vi "OutputSwerveDrive.vi"() -> ()   [LabVIEW 2020]
doc: "This VI runs feedback and feedforward controllers, manages safety interlocks, and sends commands to the swerve drive motors. This VI also controls the commanded drive shifter (low gear or high gear) state."
uses:
  <vilib>/Rock Robotics/WPI/DriverStation/WPI_DriverStationRobotMode2.ctl
  <vilib>/Rock Robotics/WPI/Solenoid/WPI_SolenoidValue.ctl
  <vilib>/Rock Robotics/WPI/ThirdParty/Phoenix-LabVIEW/Motor Controller/Controls/CTRE_Phoenix_MotorControl_ControlMode.ctl
  <vilib>/Rock Robotics/WPI/ThirdParty/Phoenix-LabVIEW/Motor Controller/Controls/CTRE_Phoenix_MotorControl_NeutralMode.ctl
  9914bed3-0d1c-4b06-b050-22aab9a27a8c.vi
  21d1f6ed-8aa7-4c08-a7f4-4e12b9ae70b2.vi
  bd7bff45-d105-4c72-b52f-b7d898b15bf8.vi
  96bdb372-2377-4471-891f-ae36cd8cf6e7.vi
  4a6563c0-2600-4cc4-b814-5bfdd37bee33.vi
  59edaa1e-6d55-4e0d-9ccd-6771bdd34e38.vi
  9422521f-1ab3-4d1d-a0e1-edf0c1a6602b.vi
  164a13db-b17b-4981-8c2b-304dea5fbafc.vi
  bf4fe2dc-b12c-4808-b801-08a1d6a94233.vi
  dd2354c2-df0e-4340-ba82-09bb2e9cf5c3.vi
  13dda775-fe22-4909-989b-e16af49b0f34.vi
  2fe6b0e9-d121-4a66-8d55-455f8b7e1020.vi
  e77e916c-e179-4e89-92bf-a3cab155e43b.vi
  sensordata.vi
  robotoutputs.vi
  GlobalDriverStationData.vi
  GlobalAutonomous.vi
  GlobalDrivebase.vi
  GRNF_CTREMotor.vi
  <vilib>/Rock Robotics/WPI/ThirdParty/Phoenix-LabVIEW/Motor Controller/Get/CTRE_Phoenix_MotorController_GetSelectedSensorData.vi
  TAI_Solenoid.vi
  GRNF_GenericSolenoid.vi
  <vilib>/Rock Robotics/WPI/Solenoid/WPI_SolenoidSetEnum.vi
  TAI_Motor.vi
panel:
  in  "Slew Rate When Slow (/s)":dbl=1.0
  in  "Slew Rate When Fast (/s)":dbl=0.8
  in  "Force to Low Gear":bool
  in  "Force To High Gear":bool
  in  "Drive Command Override [0,1]":dbl min=0.0 max=1.0 step=0.1
  in  "Manually Override Drive Calibration":bool
  in  "Time Below Speed (ms)":u32=150
  in  "Time Above Speed (ms)":u32=150
  in  "Switch to Low Gear (rpm)":dbl=1000.0
  in  "Switch to High Gear (rpm)":dbl=3500.0
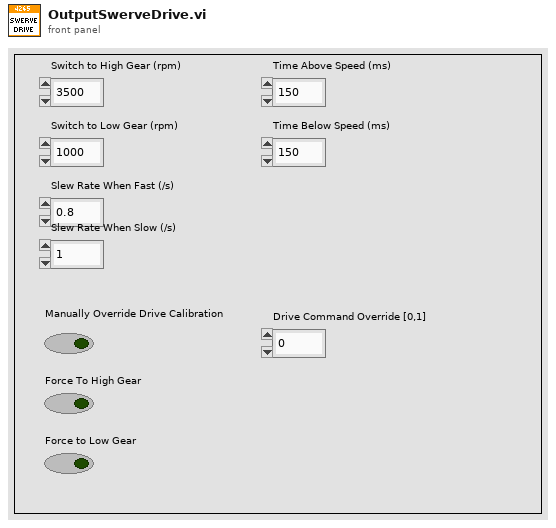
[diagram p1: front panel]
types:
  T1 = typedef "WPI_DriverStationRobotMode2.ctl" = enum16{"Autonomous Disabled", "Autonomous Enabled", "Teleop Disabled", "Teleop Enabled", "Disconnected", "Finish", "Test Disabled", "Test Enabled", "Emergency Stopped"}
  T2 = typedef "WPI_MotorControlDeviceRef.ctl" = cluster{"DeviceStatus":errorcluster, "Type":T3, "PWM":cluster{"PWM Channel":T4, "DeadBand":T5}, "CAN":cluster{"Device Number":u8, "SetOutput VI Ref":variant, "GetOutput VI Ref":variant, "Enable VI Ref":variant, "Disable VI Ref":variant, "Data":variant}, "Invert":bool, "DIO PWM":cluster{"PWM \"Enable\" Channel":T4, "DIOChannel":T6, "PWM Rate":dbl}}
  T3 = typedef "WPI_MotorControlType.ctl" = enum16{"PWM", "CAN", "DIO PWM"}
  T4 = typedef "FPGA_DIOPWMChannel.ctl" = enum8{"PWM 0", "PWM 1", "PWM 2", "PWM 3", "PWM 4", "PWM 5", "PWM 6", "PWM 7", "PWM 8", "PWM 9", "PWM MXP 0", "PWM MXP 1", "PWM MXP 2", "PWM MXP 3", "PWM MXP 4", "PWM MXP 5", "PWM MXP 6", "PWM MXP 7", "PWM MXP 8", "PWM MXP 9", "Invalid"}
  T5 = typedef "WPI_PWMDeadband.ctl" = cluster{"Name":string, "maxPositivePwm":i32, "minPositivePwm":i32, "centerPwm":i32, "maxNegativePwm":i32, "minNegativePwm":i32, "angularRange":u16}
  T6 = typedef "FPGA_DIOChannel.ctl" = enum8{"DIO 0", "DIO 1", "DIO 2", "DIO 3", "DIO 4", "DIO 5", "DIO 6", "DIO 7", "DIO 8", "DIO 9", "DIO MXP 0", "DIO MXP 1", "DIO MXP 2", "DIO MXP 3", "DIO MXP 4", "DIO MXP 5", "DIO MXP 6", "DIO MXP 7", "DIO MXP 8", "DIO MXP 9", "DIO MXP 10", "DIO MXP 11", "DIO MXP 12", "DIO MXP 13", "DIO MXP 14", "DIO MXP 15", "SPI Port CS1", "SPI Port CS2", "SPI Port CS3", "SPI Port MISO", "SPI Port MOSI", "Invalid"}
  T7 = enum16{"Low Gear", "High Gear", "Transiting", "Unknown", "Force Low Gear"}
  T8 = typedef "CTRE_Phoenix_MotorControl_NeutralMode.ctl" = enum8{"EEPROMSetting", "Override to Coast", "Override to Brake"}
  T9 = typedef "CTRE_Phoenix_MotorControl_ControlMode.ctl" = u16
  T10 = enum16{"No Changed Output", "New Normal Output", "New Testing Output"}
  T11 = typedef "WPI_SolenoidDevRef.ctl" = cluster{"DevStatus":errorcluster, "Pneumatics Control Module":u8, "Forward Solenoid Channel":T12, "Reverse Solenoid Channel":T12}
  T12 = typedef "WPI_SolenoidChannel.ctl" = enum8{"Solenoid 0", "Solenoid 1", "Solenoid 2", "Solenoid 3", "Solenoid 4", "Solenoid 5", "Solenoid 6", "Solenoid 7", "Solenoid 8", "Solenoid 9", "Solenoid 10", "Solenoid 11", "Solenoid 12", "Solenoid 13", "Solenoid 14", "Solenoid 15", "Invalid"}
  T13 = typedef "WPI_SolenoidValue.ctl" = enum16{"Off", "On", "Forward", "Reverse"}
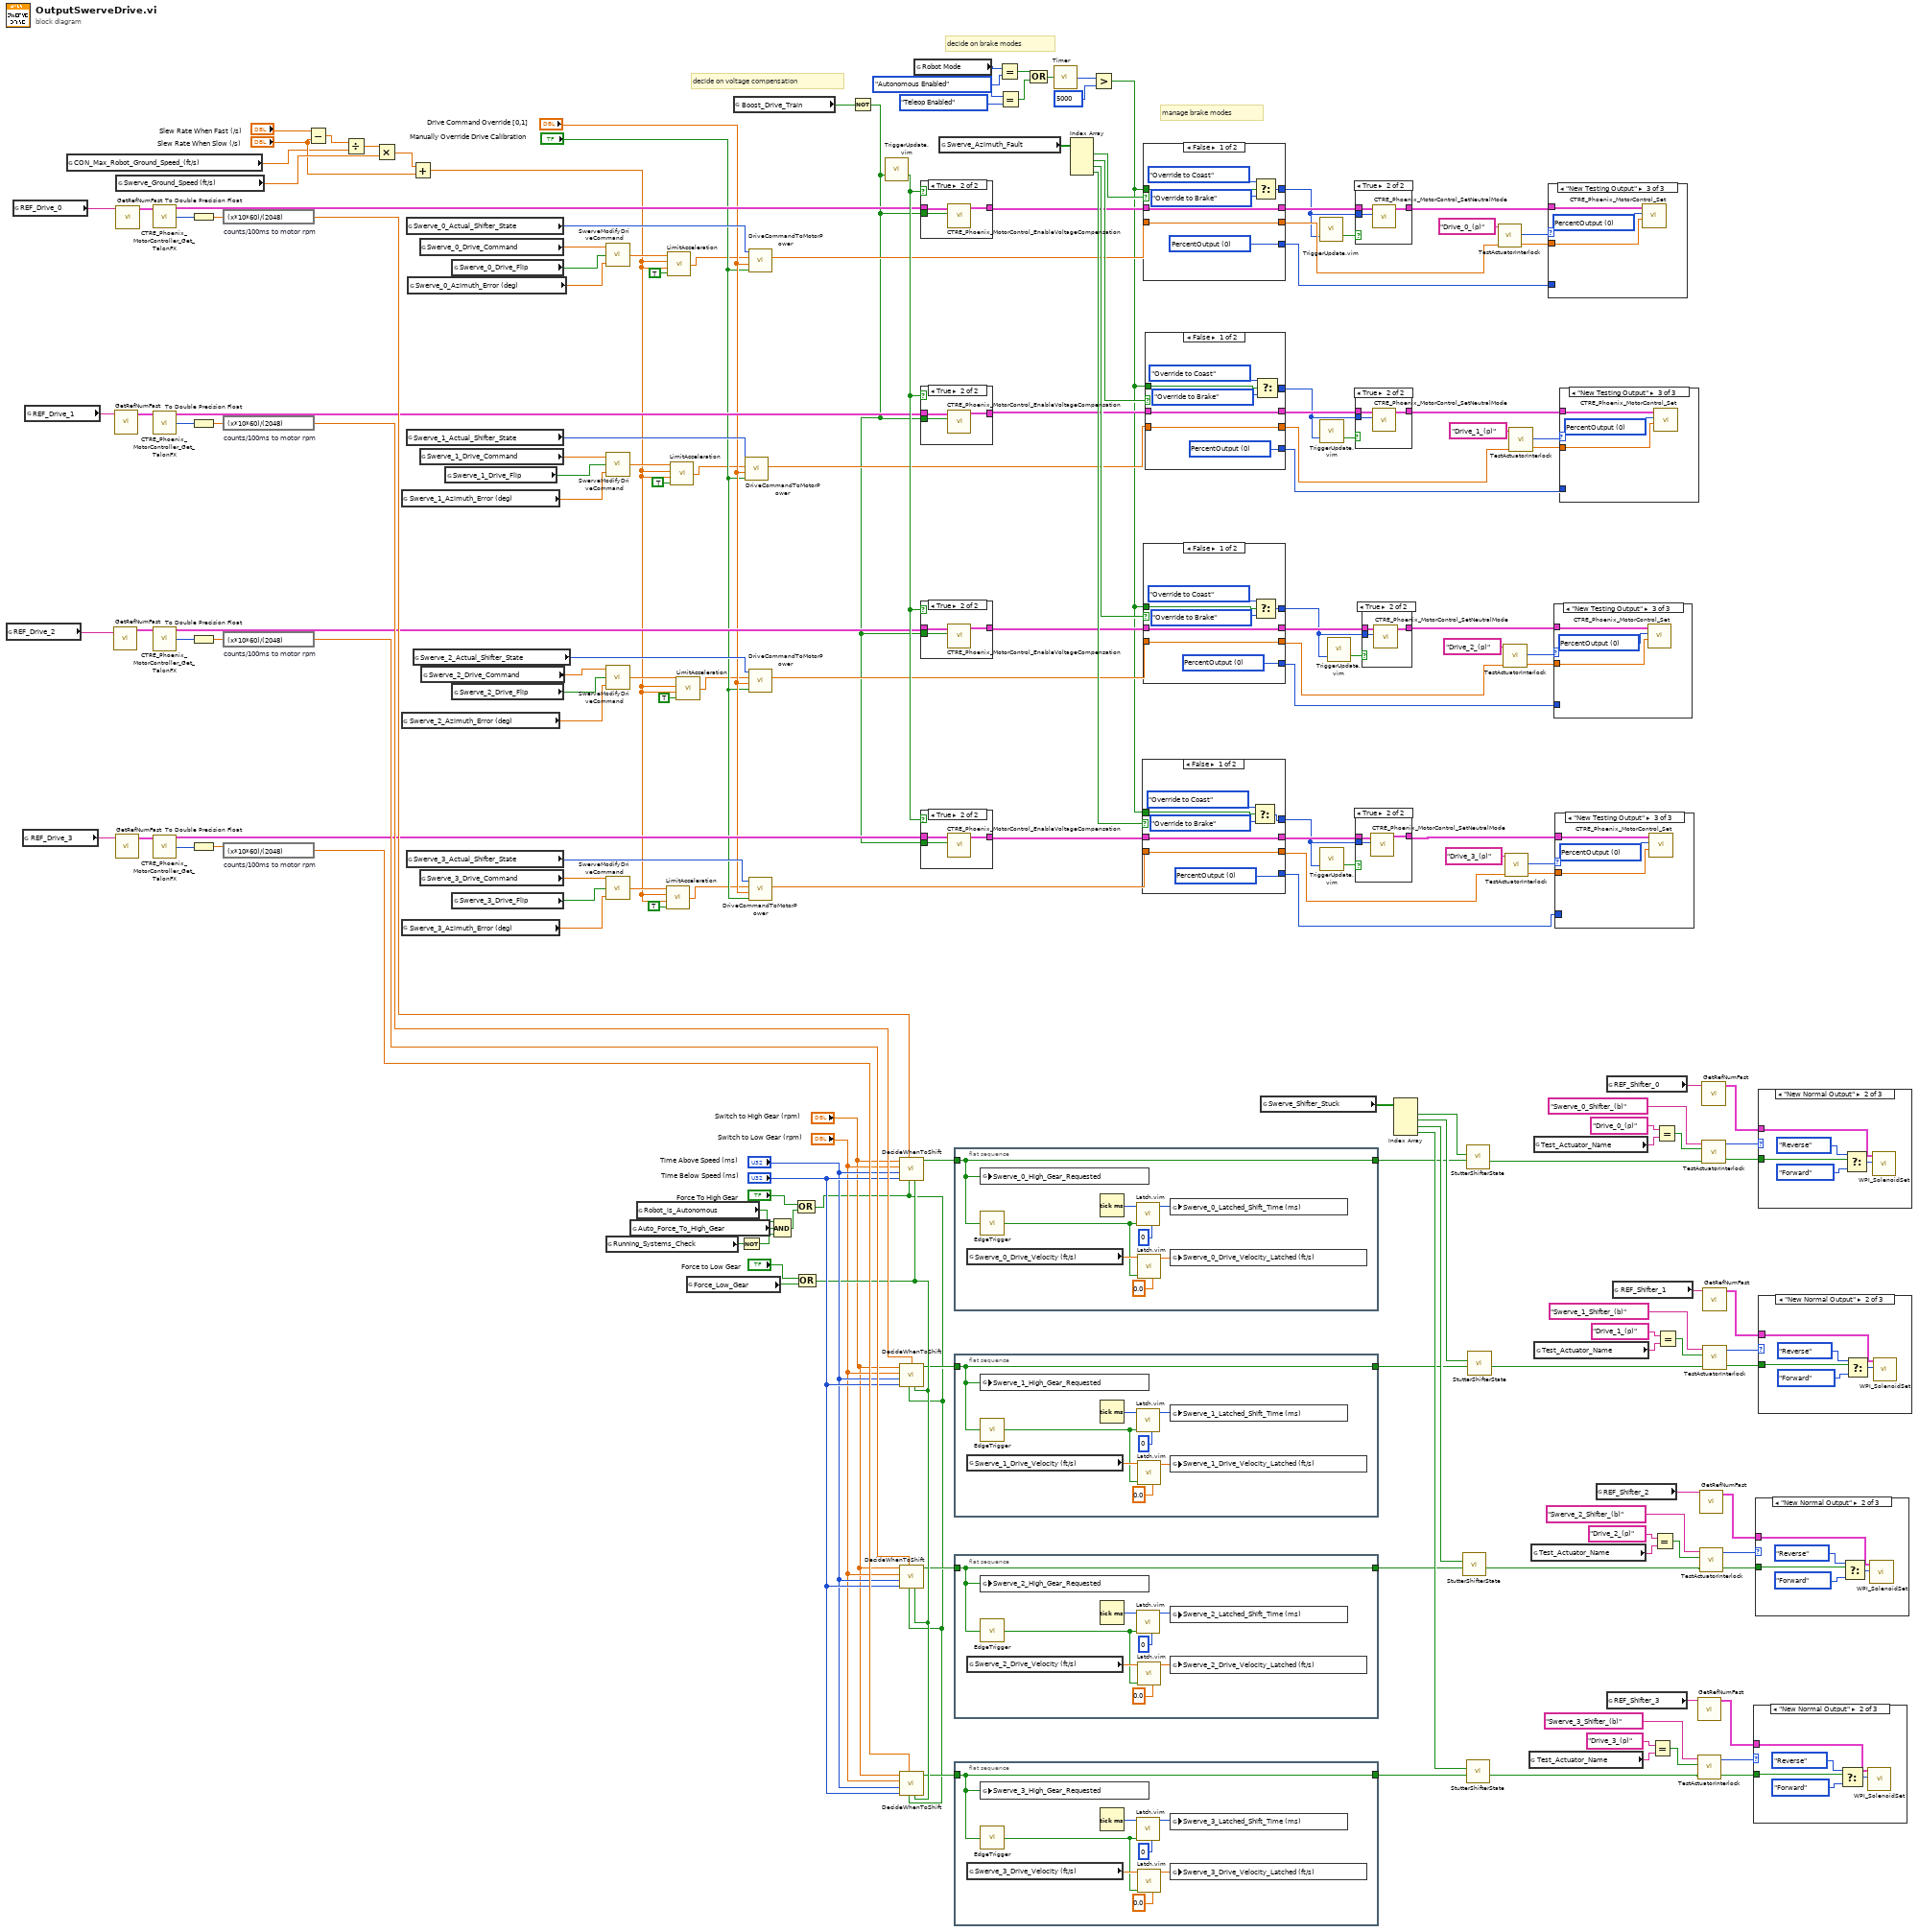
[diagram p0: block diagram]
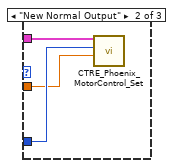
[diagram p3: hidden frame]
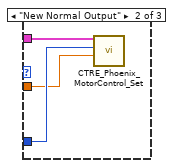
[diagram p5: hidden frame]
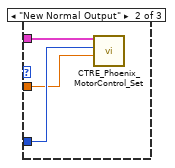
[diagram p7: hidden frame]
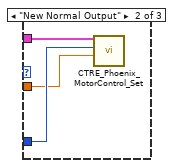
[diagram p9: hidden frame]
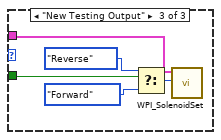
[diagram p11: hidden frame]
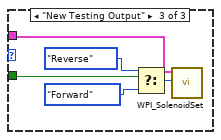
[diagram p13: hidden frame]
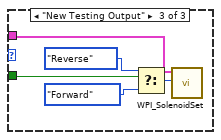
[diagram p15: hidden frame]
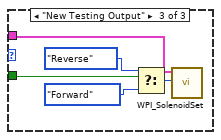
[diagram p17: hidden frame]
diagram:
  # "decide on voltage compensation"
  # "decide on brake modes"
  # "manage brake modes"
  n1 = global read "GlobalDrivebase.vi" "REF_Drive_2"() -> (w7:string)
  n2 = global read "GlobalDrivebase.vi" "REF_Drive_0"() -> (w9:string)
  n3 = global read "GlobalDrivebase.vi" "REF_Drive_3"() -> (w6:string)
  n4 = global read "GlobalDrivebase.vi" "REF_Drive_1"() -> (w8:string)
  n5 = global read "GlobalDrivebase.vi" "CON_Max_Robot_Ground_Speed_(ft/s)"() -> (w1:dbl)
  n6 = call-poly "GetRefNumFast.vi"("RefNum Name"=w7) -> ("Device Reference"=w161:T2)  [unwired: 5 in, 1 out]
  n7 = call-poly "GetRefNumFast.vi"("RefNum Name"=w8) -> ("Device Reference"=w162:T2)  [unwired: 5 in, 1 out]
  n8 = call-poly "GetRefNumFast.vi"("RefNum Name"=w6) -> ("Device Reference"=w160:T2)  [unwired: 5 in, 1 out]
  n9 = global read "sensordata.vi" "Swerve_Ground_Speed (ft/s)"() -> (w35:dbl)
  n10 = call-poly "GetRefNumFast.vi"("RefNum Name"=w9) -> ("Device Reference"=w163:T2)  [unwired: 5 in, 1 out]
  n11 = call-poly <vilib>:"CTRE_Phoenix_MotorController_Get_TalonFX.vi"("PhoenixMotorControlDevRef"=w163) -> ("PhoenixMotorControlDevRef"=w166:T2, "Velocity (Raw Sensor Units per 100 ms)"=w170:i32)  [unwired: 11 in, 2 out]
  n12 = call-poly <vilib>:"CTRE_Phoenix_MotorController_Get_TalonFX.vi"("PhoenixMotorControlDevRef"=w162) -> ("PhoenixMotorControlDevRef"=w164:T2, "Velocity (Raw Sensor Units per 100 ms)"=w169:i32)  [unwired: 11 in, 2 out]
  n13 = call-poly <vilib>:"CTRE_Phoenix_MotorController_Get_TalonFX.vi"("PhoenixMotorControlDevRef"=w161) -> ("PhoenixMotorControlDevRef"=w165:T2, "Velocity (Raw Sensor Units per 100 ms)"=w168:i32)  [unwired: 11 in, 2 out]
  n14 = call-poly <vilib>:"CTRE_Phoenix_MotorController_Get_TalonFX.vi"("PhoenixMotorControlDevRef"=w160) -> ("PhoenixMotorControlDevRef"=w155:T2, "Velocity (Raw Sensor Units per 100 ms)"=w167:i32)  [unwired: 11 in, 2 out]
  n15 = To Double Precision Float(number=w170) -> (double precision float=w177:dbl)
  n16 = To Double Precision Float(number=w169) -> (double precision float=w176:dbl)
  n17 = To Double Precision Float(number=w168) -> (double precision float=w175:dbl)
  n18 = To Double Precision Float(number=w167) -> (double precision float=w174:dbl)
  n19 = expression code="(x*10*60)/(2048)" "counts/100ms to motor rpm"(w177) -> (w171:dbl)
  n20 = expression code="(x*10*60)/(2048)" "counts/100ms to motor rpm"(w176) -> (w172:dbl)
  n21 = expression code="(x*10*60)/(2048)" "counts/100ms to motor rpm"(w175) -> (w173:dbl)
  n22 = expression code="(x*10*60)/(2048)" "counts/100ms to motor rpm"(w174) -> (w179:dbl)
  n23 = Subtract(x="Slew Rate When Fast (/s)", y="Slew Rate When Slow (/s)") -> (x-y=w37:dbl)
  n24 = Divide(x=w37, y=w1) -> (x/y=w36:dbl)
  n25 = Multiply(x=w36, y=w35) -> (x*y=w34:dbl)
  n26 = global read "robotoutputs.vi" "Swerve_1_Azimuth_Error (deg)"() -> (w28:dbl)
  n27 = global read "robotoutputs.vi" "Swerve_2_Azimuth_Error (deg)"() -> (w27:dbl)
  n28 = global read "robotoutputs.vi" "Swerve_3_Azimuth_Error (deg)"() -> (w26:dbl)
  n29 = global read "sensordata.vi" "Swerve_0_Actual_Shifter_State"() -> (w154:T7)
  n30 = global read "sensordata.vi" "Swerve_1_Actual_Shifter_State"() -> (w152:T7)
  n31 = global read "sensordata.vi" "Swerve_3_Actual_Shifter_State"() -> (w148:T7)
  n32 = global read "robotoutputs.vi" "Swerve_0_Azimuth_Error (deg)"() -> (w29:dbl)
  n33 = Add(x=w34, y="Slew Rate When Slow (/s)") -> (x+y=w32:dbl)
  n34 = global read "sensordata.vi" "Swerve_2_Actual_Shifter_State"() -> (w150:T7)
  n35 = global read "robotoutputs.vi" "Swerve_0_Drive_Command"() -> (w53:dbl)
  n36 = global read "robotoutputs.vi" "Swerve_1_Drive_Command"() -> (w54:dbl)
  n37 = global read "robotoutputs.vi" "Swerve_3_Drive_Command"() -> (w56:dbl)
  n38 = global read "robotoutputs.vi" "Swerve_2_Drive_Command"() -> (w55:dbl)
  n39 = global read "robotoutputs.vi" "Swerve_1_Drive_Flip"() -> (w143:bool)
  n40 = global read "robotoutputs.vi" "Swerve_0_Drive_Flip"() -> (w141:bool)
  n41 = global read "robotoutputs.vi" "Swerve_2_Drive_Flip"() -> (w144:bool)
  n42 = global read "robotoutputs.vi" "Swerve_3_Drive_Flip"() -> (w142:bool)
  n43 = global read "GlobalDriverStationData.vi" "Running_Systems_Check"() -> (w11:bool)
  n44 = call "SwerveModifyDriveCommand.vi"("Azimuth Error (deg)"=w29, "Flip Drive Command"=w141, "Raw Drive Command (ul)"=w53) -> ("Modified Drive Command (ul)"=w51:dbl)
  n45 = call "SwerveModifyDriveCommand.vi"("Azimuth Error (deg)"=w28, "Flip Drive Command"=w143, "Raw Drive Command (ul)"=w54) -> ("Modified Drive Command (ul)"=w49:dbl)
  n46 = call "SwerveModifyDriveCommand.vi"("Azimuth Error (deg)"=w27, "Flip Drive Command"=w144, "Raw Drive Command (ul)"=w55) -> ("Modified Drive Command (ul)"=w47:dbl)
  n47 = call "SwerveModifyDriveCommand.vi"("Azimuth Error (deg)"=w26, "Flip Drive Command"=w142, "Raw Drive Command (ul)"=w56) -> ("Modified Drive Command (ul)"=w45:dbl)
  n48 = global read "GlobalAutonomous.vi" "Auto_Force_To_High_Gear"() -> (w22:bool)
  n49 = global read "GlobalDriverStationData.vi" "Robot_is_Autonomous"() -> (w23:bool)
  n50 = call "LimitAcceleration.vi"("Apply Limit"=TRUE, "Decceleration Limit (/s)"=w32, "Acceleration Limit (/s)"=w32, "Raw Input"=w45) -> ("Output"=w44:dbl)
  n51 = call "LimitAcceleration.vi"("Apply Limit"=TRUE, "Decceleration Limit (/s)"=w32, "Acceleration Limit (/s)"=w32, "Raw Input"=w51) -> ("Output"=w50:dbl)
  n52 = call "LimitAcceleration.vi"("Apply Limit"=TRUE, "Decceleration Limit (/s)"=w32, "Acceleration Limit (/s)"=w32, "Raw Input"=w49) -> ("Output"=w48:dbl)
  n53 = call "LimitAcceleration.vi"("Apply Limit"=TRUE, "Decceleration Limit (/s)"=w32, "Acceleration Limit (/s)"=w32, "Raw Input"=w47) -> ("Output"=w46:dbl)
  n54 = global read "robotoutputs.vi" "Force_Low_Gear"() -> (w132:bool)
  n55 = global read "robotoutputs.vi" "Boost_Drive_Train"() -> (w30:bool)
  n56 = Not(x=w11) -> (.not. x?=w10:bool)
  n57 = call "DriveCommandToMotorPower.vi"("Drive Command Override"="Manually Override Drive Calibration", "Drive Command Override (ul) [-1,1]"="Drive Command Override [0,1]", "Drive Command (ul) [-1,1]"=w48, "Actual Shifter State"=w152) -> ("Motor Power (ul) [-1,1]"=w151:dbl)  [unwired: 7 in]
  n58 = call "DriveCommandToMotorPower.vi"("Drive Command Override"="Manually Override Drive Calibration", "Drive Command Override (ul) [-1,1]"="Drive Command Override [0,1]", "Drive Command (ul) [-1,1]"=w50, "Actual Shifter State"=w154) -> ("Motor Power (ul) [-1,1]"=w153:dbl)  [unwired: 7 in]
  n59 = call "DriveCommandToMotorPower.vi"("Drive Command Override"="Manually Override Drive Calibration", "Drive Command Override (ul) [-1,1]"="Drive Command Override [0,1]", "Drive Command (ul) [-1,1]"=w46, "Actual Shifter State"=w150) -> ("Motor Power (ul) [-1,1]"=w149:dbl)  [unwired: 7 in]
  n60 = call "DriveCommandToMotorPower.vi"("Drive Command Override"="Manually Override Drive Calibration", "Drive Command Override (ul) [-1,1]"="Drive Command Override [0,1]", "Drive Command (ul) [-1,1]"=w44, "Actual Shifter State"=w148) -> ("Motor Power (ul) [-1,1]"=w147:dbl)  [unwired: 7 in]
  n61 = Compound Arithmetic op=AND(w23, w22, w10) -> (w21:bool)
  n62 = Compound Arithmetic op=OR("Force To High Gear", w21) -> (w24:bool)
  n63 = Compound Arithmetic op=OR("Force to Low Gear", w132) -> (w133:bool)
  n64 = Not(x=w30) -> (.not. x?=w31:bool)
  n65 = call "TriggerUpdate.vim"("Trigger"=w31) -> ("Update"=w178:bool)  [unwired: 2 in]
  n66 = call "DecideWhenToShift.vi"("Force to Low Gear"=w133, "Force To High Gear"=w24, "Drive Motor Speed (rpm)"=w171, "Time Below Speed (ms)"="Time Below Speed (ms)", "Time Above Speed (ms)"="Time Above Speed (ms)", "Switch to Low Gear (rpm)"="Switch to Low Gear (rpm)", "Switch to High Gear (rpm)"="Switch to High Gear (rpm)") -> ("Requested Shifter State"=w122:bool)  [unwired: 4 in]
  n67 = call "DecideWhenToShift.vi"("Force to Low Gear"=w133, "Force To High Gear"=w24, "Drive Motor Speed (rpm)"=w172, "Time Below Speed (ms)"="Time Below Speed (ms)", "Time Above Speed (ms)"="Time Above Speed (ms)", "Switch to Low Gear (rpm)"="Switch to Low Gear (rpm)", "Switch to High Gear (rpm)"="Switch to High Gear (rpm)") -> ("Requested Shifter State"=w120:bool)  [unwired: 4 in]
  n68 = call "DecideWhenToShift.vi"("Force to Low Gear"=w133, "Force To High Gear"=w24, "Drive Motor Speed (rpm)"=w173, "Time Below Speed (ms)"="Time Below Speed (ms)", "Time Above Speed (ms)"="Time Above Speed (ms)", "Switch to Low Gear (rpm)"="Switch to Low Gear (rpm)", "Switch to High Gear (rpm)"="Switch to High Gear (rpm)") -> ("Requested Shifter State"=w118:bool)  [unwired: 4 in]
  n69 = call "DecideWhenToShift.vi"("Force to Low Gear"=w133, "Force To High Gear"=w24, "Drive Motor Speed (rpm)"=w179, "Time Below Speed (ms)"="Time Below Speed (ms)", "Time Above Speed (ms)"="Time Above Speed (ms)", "Switch to Low Gear (rpm)"="Switch to Low Gear (rpm)", "Switch to High Gear (rpm)"="Switch to High Gear (rpm)") -> ("Requested Shifter State"=w116:bool)  [unwired: 4 in]
  n70 = global read "GlobalDriverStationData.vi" "Robot Mode"() -> (w16:T1)
  n71 = case shown="True" w178 {
    tunnel: w166 -> [w187 w190]
    tunnel: [w187 w189] -> w159
    tunnel: w31 -> [_ w188]
    frame False {
    }
    frame True {
      n72 = call <vilib>:"CTRE_Phoenix_MotorControl_EnableVoltageCompensation.vi"("Enable Voltage Compensation?"=w188, "PhoenixMotorControlDevRef"=w190) -> ("PhoenixMotorControlDevRef"=w189:T2)  [unwired: 8 in, 1 out]
    }
  }
  n73 = case shown="True" w178 {
    tunnel: w164 -> [w191 w194]
    tunnel: [w191 w193] -> w158
    tunnel: w31 -> [_ w192]
    frame False {
    }
    frame True {
      n74 = call <vilib>:"CTRE_Phoenix_MotorControl_EnableVoltageCompensation.vi"("Enable Voltage Compensation?"=w192, "PhoenixMotorControlDevRef"=w194) -> ("PhoenixMotorControlDevRef"=w193:T2)  [unwired: 8 in, 1 out]
    }
  }
  n75 = case shown="True" w178 {
    tunnel: w165 -> [w195 w198]
    tunnel: [w195 w197] -> w157
    tunnel: w31 -> [_ w196]
    frame False {
    }
    frame True {
      n76 = call <vilib>:"CTRE_Phoenix_MotorControl_EnableVoltageCompensation.vi"("Enable Voltage Compensation?"=w196, "PhoenixMotorControlDevRef"=w198) -> ("PhoenixMotorControlDevRef"=w197:T2)  [unwired: 8 in, 1 out]
    }
  }
  n77 = case shown="True" w178 {
    tunnel: [w199 w202] -> w156
    tunnel: w31 -> [_ w201]
    tunnel: w155 -> [w199 w200]
    frame False {
    }
    frame True {
      n78 = call <vilib>:"CTRE_Phoenix_MotorControl_EnableVoltageCompensation.vi"("Enable Voltage Compensation?"=w201, "PhoenixMotorControlDevRef"=w200) -> ("PhoenixMotorControlDevRef"=w202:T2)  [unwired: 8 in, 1 out]
    }
  }
  n79 = global read "sensordata.vi" "Swerve_Azimuth_Fault"() -> (w186:bool[])
  n80 = flat-sequence {
    tunnel: w122 -> [w210]
    tunnel: [w210] -> w121
    frame #0 {
      n81 = global read "sensordata.vi" "Swerve_0_Drive_Velocity (ft/s)"() -> (w207:dbl)
      n82 = global write "robotoutputs.vi" "Swerve_0_High_Gear_Requested"(w210) -> ()
      n83 = call "EdgeTrigger.vi"("Input Signal"=w210) -> ("All Edge Trigger"=w205:bool)  [unwired: 2 out]
      n84 = Tick Count (ms)() -> (millisecond timer value=w209:u32)
      n85 = call "Latch.vim"("Default Value"=u32 0 ("millisecond timer value"), "Latch Signal"=w205, "Latch Value"=w209) -> ("Latched"=w203:u32)  [unwired: 8 in]
      n86 = call "Latch.vim"("Default Value"=0.0, "Latch Signal"=w205, "Latch Value"=w207) -> ("Latched"=w204:dbl)  [unwired: 8 in]
      n87 = global write "sensordata.vi" "Swerve_0_Latched_Shift_Time (ms)"(w203) -> ()
      n88 = global write "sensordata.vi" "Swerve_0_Drive_Velocity_Latched (ft/s)"(w204) -> ()
    }
  }
  n89 = flat-sequence {
    tunnel: w120 -> [w218]
    tunnel: [w218] -> w119
    frame #0 {
      n90 = global read "sensordata.vi" "Swerve_1_Drive_Velocity (ft/s)"() -> (w215:dbl)
      n91 = global write "robotoutputs.vi" "Swerve_1_High_Gear_Requested"(w218) -> ()
      n92 = call "EdgeTrigger.vi"("Input Signal"=w218) -> ("All Edge Trigger"=w213:bool)  [unwired: 2 out]
      n93 = Tick Count (ms)() -> (millisecond timer value=w217:u32)
      n94 = call "Latch.vim"("Default Value"=u32 0 ("millisecond timer value"), "Latch Signal"=w213, "Latch Value"=w217) -> ("Latched"=w211:u32)  [unwired: 8 in]
      n95 = call "Latch.vim"("Default Value"=0.0, "Latch Signal"=w213, "Latch Value"=w215) -> ("Latched"=w212:dbl)  [unwired: 8 in]
      n96 = global write "sensordata.vi" "Swerve_1_Latched_Shift_Time (ms)"(w211) -> ()
      n97 = global write "sensordata.vi" "Swerve_1_Drive_Velocity_Latched (ft/s)"(w212) -> ()
    }
  }
  n98 = flat-sequence {
    tunnel: w118 -> [w226]
    tunnel: [w226] -> w117
    frame #0 {
      n99 = global read "sensordata.vi" "Swerve_2_Drive_Velocity (ft/s)"() -> (w223:dbl)
      n100 = global write "robotoutputs.vi" "Swerve_2_High_Gear_Requested"(w226) -> ()
      n101 = call "EdgeTrigger.vi"("Input Signal"=w226) -> ("All Edge Trigger"=w221:bool)  [unwired: 2 out]
      n102 = Tick Count (ms)() -> (millisecond timer value=w225:u32)
      n103 = call "Latch.vim"("Default Value"=u32 0 ("millisecond timer value"), "Latch Signal"=w221, "Latch Value"=w225) -> ("Latched"=w219:u32)  [unwired: 8 in]
      n104 = call "Latch.vim"("Default Value"=0.0, "Latch Signal"=w221, "Latch Value"=w223) -> ("Latched"=w220:dbl)  [unwired: 8 in]
      n105 = global write "sensordata.vi" "Swerve_2_Latched_Shift_Time (ms)"(w219) -> ()
      n106 = global write "sensordata.vi" "Swerve_2_Drive_Velocity_Latched (ft/s)"(w220) -> ()
    }
  }
  n107 = flat-sequence {
    tunnel: w116 -> [w234]
    tunnel: [w234] -> w115
    frame #0 {
      n108 = global read "sensordata.vi" "Swerve_3_Drive_Velocity (ft/s)"() -> (w231:dbl)
      n109 = global write "robotoutputs.vi" "Swerve_3_High_Gear_Requested"(w234) -> ()
      n110 = call "EdgeTrigger.vi"("Input Signal"=w234) -> ("All Edge Trigger"=w229:bool)  [unwired: 2 out]
      n111 = Tick Count (ms)() -> (millisecond timer value=w233:u32)
      n112 = call "Latch.vim"("Default Value"=u32 0 ("millisecond timer value"), "Latch Signal"=w229, "Latch Value"=w233) -> ("Latched"=w227:u32)  [unwired: 8 in]
      n113 = call "Latch.vim"("Default Value"=0.0, "Latch Signal"=w229, "Latch Value"=w231) -> ("Latched"=w228:dbl)  [unwired: 8 in]
      n114 = global write "sensordata.vi" "Swerve_3_Latched_Shift_Time (ms)"(w227) -> ()
      n115 = global write "sensordata.vi" "Swerve_3_Drive_Velocity_Latched (ft/s)"(w228) -> ()
    }
  }
  n116 = Equal?(x=w16, y=WPI_DriverStationRobotMode2."Autonomous Enabled" ("Robot Mode")) -> (x = y?=w20:bool)
  n117 = Equal?(x=w16, y=WPI_DriverStationRobotMode2."Teleop Enabled") -> (x = y?=w19:bool)
  n118 = Compound Arithmetic op=OR(w20, w19) -> (w15:bool)
  n119 = call "Timer.vi"("Reset Timer"=w15) -> ("Time (ms)"=w14:u32)
  n120 = Index Array(array=w186) -> (element #1=w182:bool, element #2=w181:bool, element #3=w180:bool, element #4=w185:bool)  [unwired: 4 in]
  n121 = Greater?(x=w14, y=u32 5000) -> (0:w12:bool)
  n122 = case shown="False" w185 {
    tunnel: [w241 w245] -> w123
    tunnel: w156 -> [w241 w245]
    tunnel: [w240 0.0 ("Command")] -> w62
    tunnel: w147 -> [w240 _]
    tunnel: [w239 w243] -> w61
    tunnel: [w236 CTRE_Phoenix_MotorControl_NeutralMode."Override to Coast" ("Motor Control Neutral Mode")] -> w107
    tunnel: w12 -> [w235 _]
    frame False {
      w239 = T9 0 items=["PercentOutput"=0, "Position"=1, "Velocity"=2, "Current"=3, "Follower"=5, "MotionProfile"=6, "MotionMagic"=7, "MotionProfileArc"=10, "Disabled"=15] ("Control Mode")
      n123 = Select(t=CTRE_Phoenix_MotorControl_NeutralMode."Override to Coast" ("Motor Control Neutral Mode"), s=w235, f=CTRE_Phoenix_MotorControl_NeutralMode."Override to Brake" ("Motor Control Neutral Mode")) -> (s? t:f=w236:T8)
    }
    frame True {
      w243 = T9 0 items=["PercentOutput"=0, "Position"=1, "Velocity"=2, "Current"=3, "Follower"=5, "MotionProfile"=6, "MotionMagic"=7, "MotionProfileArc"=10, "Disabled"=15] ("Control Mode")
    }
  }
  n124 = case shown="False" w182 {
    tunnel: [w252 w256] -> w126
    tunnel: w159 -> [w252 w256]
    tunnel: [w251 0.0 ("Command")] -> w183
    tunnel: w153 -> [w251 _]
    tunnel: [w250 w254] -> w80
    tunnel: [w248 CTRE_Phoenix_MotorControl_NeutralMode."Override to Coast" ("Motor Control Neutral Mode")] -> w114
    tunnel: w12 -> [w246 _]
    frame False {
      w250 = T9 0 items=["PercentOutput"=0, "Position"=1, "Velocity"=2, "Current"=3, "Follower"=5, "MotionProfile"=6, "MotionMagic"=7, "MotionProfileArc"=10, "Disabled"=15] ("Control Mode")
      n125 = Select(t=CTRE_Phoenix_MotorControl_NeutralMode."Override to Coast" ("Motor Control Neutral Mode"), s=w246, f=CTRE_Phoenix_MotorControl_NeutralMode."Override to Brake" ("Motor Control Neutral Mode")) -> (s? t:f=w248:T8)
    }
    frame True {
      w254 = T9 0 items=["PercentOutput"=0, "Position"=1, "Velocity"=2, "Current"=3, "Follower"=5, "MotionProfile"=6, "MotionMagic"=7, "MotionProfileArc"=10, "Disabled"=15] ("Control Mode")
    }
  }
  n126 = case shown="False" w180 {
    tunnel: [w263 w267] -> w124
    tunnel: w157 -> [w263 w267]
    tunnel: [w262 0.0 ("Command")] -> w68
    tunnel: w149 -> [w262 _]
    tunnel: [w261 w265] -> w67
    tunnel: [w258 CTRE_Phoenix_MotorControl_NeutralMode."Override to Coast" ("Motor Control Neutral Mode")] -> w109
    tunnel: w12 -> [w257 _]
    frame False {
      w261 = T9 0 items=["PercentOutput"=0, "Position"=1, "Velocity"=2, "Current"=3, "Follower"=5, "MotionProfile"=6, "MotionMagic"=7, "MotionProfileArc"=10, "Disabled"=15] ("Control Mode")
      n127 = Select(t=CTRE_Phoenix_MotorControl_NeutralMode."Override to Coast" ("Motor Control Neutral Mode"), s=w257, f=CTRE_Phoenix_MotorControl_NeutralMode."Override to Brake" ("Motor Control Neutral Mode")) -> (s? t:f=w258:T8)
    }
    frame True {
      w265 = T9 0 items=["PercentOutput"=0, "Position"=1, "Velocity"=2, "Current"=3, "Follower"=5, "MotionProfile"=6, "MotionMagic"=7, "MotionProfileArc"=10, "Disabled"=15] ("Control Mode")
    }
  }
  n128 = case shown="False" w181 {
    tunnel: [w274 w278] -> w125
    tunnel: w158 -> [w274 w278]
    tunnel: [w273 0.0 ("Command")] -> w75
    tunnel: w151 -> [w273 _]
    tunnel: [w272 w276] -> w74
    tunnel: [w269 CTRE_Phoenix_MotorControl_NeutralMode."Override to Coast" ("Motor Control Neutral Mode")] -> w112
    tunnel: w12 -> [w268 _]
    frame False {
      w272 = T9 0 items=["PercentOutput"=0, "Position"=1, "Velocity"=2, "Current"=3, "Follower"=5, "MotionProfile"=6, "MotionMagic"=7, "MotionProfileArc"=10, "Disabled"=15] ("Control Mode")
      n129 = Select(t=CTRE_Phoenix_MotorControl_NeutralMode."Override to Coast" ("Motor Control Neutral Mode"), s=w268, f=CTRE_Phoenix_MotorControl_NeutralMode."Override to Brake" ("Motor Control Neutral Mode")) -> (s? t:f=w269:T8)
    }
    frame True {
      w276 = T9 0 items=["PercentOutput"=0, "Position"=1, "Velocity"=2, "Current"=3, "Follower"=5, "MotionProfile"=6, "MotionMagic"=7, "MotionProfileArc"=10, "Disabled"=15] ("Control Mode")
    }
  }
  n130 = global read "sensordata.vi" "Swerve_Shifter_Stuck"() -> (w131:bool[])
  n131 = call "TriggerUpdate.vim"("Trigger"=w114) -> ("Update"=w113:bool)  [unwired: 2 in]
  n132 = call "TriggerUpdate.vim"("Trigger"=w112) -> ("Update"=w111:bool)  [unwired: 2 in]
  n133 = call "TriggerUpdate.vim"("Trigger"=w107) -> ("Update"=w108:bool)  [unwired: 2 in]
  n134 = call "TriggerUpdate.vim"("Trigger"=w109) -> ("Update"=w110:bool)  [unwired: 2 in]
  n135 = case shown="True" w111 {
    tunnel: w125 -> [w279 w282]
    tunnel: [w279 w281] -> w73
    tunnel: w112 -> [_ w280]
    frame False {
    }
    frame True {
      n136 = call <vilib>:"CTRE_Phoenix_MotorControl_SetNeutralMode.vi"("Motor Control Neutral Mode"=w280, "PhoenixMotorControlDevRef"=w282) -> ("PhoenixMotorControlDevRef"=w281:T2)  [unwired: 8 in, 1 out]
    }
  }
  n137 = case shown="True" w113 {
    tunnel: w114 -> [_ w286]
    tunnel: w126 -> [w283 w285]
    tunnel: [w283 w284] -> w79
    frame False {
    }
    frame True {
      n138 = call <vilib>:"CTRE_Phoenix_MotorControl_SetNeutralMode.vi"("Motor Control Neutral Mode"=w286, "PhoenixMotorControlDevRef"=w285) -> ("PhoenixMotorControlDevRef"=w284:T2)  [unwired: 8 in, 1 out]
    }
  }
  n139 = case shown="True" w108 {
    tunnel: w123 -> [w287 w290]
    tunnel: [w287 w289] -> w63
    tunnel: w107 -> [_ w288]
    frame False {
    }
    frame True {
      n140 = call <vilib>:"CTRE_Phoenix_MotorControl_SetNeutralMode.vi"("Motor Control Neutral Mode"=w288, "PhoenixMotorControlDevRef"=w290) -> ("PhoenixMotorControlDevRef"=w289:T2)  [unwired: 8 in, 1 out]
    }
  }
  n141 = case shown="True" w110 {
    tunnel: w124 -> [w291 w294]
    tunnel: [w291 w293] -> w69
    tunnel: w109 -> [_ w292]
    frame False {
    }
    frame True {
      n142 = call <vilib>:"CTRE_Phoenix_MotorControl_SetNeutralMode.vi"("Motor Control Neutral Mode"=w292, "PhoenixMotorControlDevRef"=w294) -> ("PhoenixMotorControlDevRef"=w293:T2)  [unwired: 8 in, 1 out]
    }
  }
  n143 = Index Array(array=w131) -> (element #1=w130:bool, element #2=w129:bool, element #3=w128:bool, element #4=w127:bool)  [unwired: 4 in]
  n144 = call "StutterShifterState.vi"("Requested Shifter State"=w117, "Request Stutter"=w128) -> ("Stuttered Shifter State"=w58:bool)  [unwired: 9 in]
  n145 = call "StutterShifterState.vi"("Requested Shifter State"=w121, "Request Stutter"=w130) -> ("Stuttered Shifter State"=w60:bool)  [unwired: 9 in]
  n146 = call "StutterShifterState.vi"("Requested Shifter State"=w115, "Request Stutter"=w127) -> ("Stuttered Shifter State"=w57:bool)  [unwired: 9 in]
  n147 = call "StutterShifterState.vi"("Requested Shifter State"=w119, "Request Stutter"=w129) -> ("Stuttered Shifter State"=w59:bool)  [unwired: 9 in]
  n148 = call-poly "TestActuatorInterlock.vi"("Normal Output"=w183, "Actuator Name"="Drive_0_(p)" ("Actuator_Name")) -> ("Interlocked Output"=w39:dbl, "Output Mode"=w81:T10)  [unwired: 3 in]
  n149 = call-poly "TestActuatorInterlock.vi"("Normal Output"=w68, "Actuator Name"="Drive_2_(p)" ("Actuator_Name")) -> ("Interlocked Output"=w70:dbl, "Output Mode"=w71:T10)  [unwired: 3 in]
  n150 = call-poly "TestActuatorInterlock.vi"("Normal Output"=w62, "Actuator Name"="Drive_3_(p)" ("Actuator_Name")) -> ("Interlocked Output"=w64:dbl, "Output Mode"=w65:T10)  [unwired: 3 in]
  n151 = call-poly "TestActuatorInterlock.vi"("Normal Output"=w75, "Actuator Name"="Drive_1_(p)" ("Actuator_Name")) -> ("Interlocked Output"=w76:dbl, "Output Mode"=w77:T10)  [unwired: 3 in]
  n152 = global read "GlobalDriverStationData.vi" "Test_Actuator_Name"() -> (w138:string)
  n153 = global read "GlobalDriverStationData.vi" "Test_Actuator_Name"() -> (w100:string)
  n154 = global read "GlobalDriverStationData.vi" "Test_Actuator_Name"() -> (w86:string)
  n155 = global read "GlobalDriverStationData.vi" "Test_Actuator_Name"() -> (w93:string)
  n156 = case shown="\"New Testing Output\"" w81 {
    tunnel: w80 -> [_ w297 _]
    tunnel: w79 -> [_ w295 w299]
    tunnel: w39 -> [_ w296 w298]
    frame "No Changed Output", Default {
    }
    frame "New Normal Output" {
      n157 = call <vilib>:"CTRE_Phoenix_MotorControl_Set.vi"("Output"=w296, "Control Mode"=w297, "PhoenixMotorControlDevRef"=w295) -> ()  [unwired: 7 in, 2 out]
    }
    frame "New Testing Output" {
      w300 = T9 0 items=["PercentOutput"=0, "Position"=1, "Velocity"=2, "Current"=3, "Follower"=5, "MotionProfile"=6, "MotionMagic"=7, "MotionProfileArc"=10, "Disabled"=15] ("Control Mode")
      n158 = call <vilib>:"CTRE_Phoenix_MotorControl_Set.vi"("Output"=w298, "Control Mode"=w300, "PhoenixMotorControlDevRef"=w299) -> ()  [unwired: 7 in, 2 out]
    }
  }
  n159 = case shown="\"New Testing Output\"" w71 {
    tunnel: w67 -> [_ w303 _]
    tunnel: w69 -> [_ w301 w305]
    tunnel: w70 -> [_ w302 w304]
    frame "No Changed Output", Default {
    }
    frame "New Normal Output" {
      n160 = call <vilib>:"CTRE_Phoenix_MotorControl_Set.vi"("Output"=w302, "Control Mode"=w303, "PhoenixMotorControlDevRef"=w301) -> ()  [unwired: 7 in, 2 out]
    }
    frame "New Testing Output" {
      w306 = T9 0 items=["PercentOutput"=0, "Position"=1, "Velocity"=2, "Current"=3, "Follower"=5, "MotionProfile"=6, "MotionMagic"=7, "MotionProfileArc"=10, "Disabled"=15] ("Control Mode")
      n161 = call <vilib>:"CTRE_Phoenix_MotorControl_Set.vi"("Output"=w304, "Control Mode"=w306, "PhoenixMotorControlDevRef"=w305) -> ()  [unwired: 7 in, 2 out]
    }
  }
  n162 = case shown="\"New Testing Output\"" w65 {
    tunnel: w61 -> [_ w309 _]
    tunnel: w63 -> [_ w307 w311]
    tunnel: w64 -> [_ w308 w310]
    frame "No Changed Output", Default {
    }
    frame "New Normal Output" {
      n163 = call <vilib>:"CTRE_Phoenix_MotorControl_Set.vi"("Output"=w308, "Control Mode"=w309, "PhoenixMotorControlDevRef"=w307) -> ()  [unwired: 7 in, 2 out]
    }
    frame "New Testing Output" {
      w312 = T9 0 items=["PercentOutput"=0, "Position"=1, "Velocity"=2, "Current"=3, "Follower"=5, "MotionProfile"=6, "MotionMagic"=7, "MotionProfileArc"=10, "Disabled"=15] ("Control Mode")
      n164 = call <vilib>:"CTRE_Phoenix_MotorControl_Set.vi"("Output"=w310, "Control Mode"=w312, "PhoenixMotorControlDevRef"=w311) -> ()  [unwired: 7 in, 2 out]
    }
  }
  n165 = case shown="\"New Testing Output\"" w77 {
    tunnel: w74 -> [_ w315 _]
    tunnel: w73 -> [_ w313 w317]
    tunnel: w76 -> [_ w314 w316]
    frame "No Changed Output", Default {
    }
    frame "New Normal Output" {
      n166 = call <vilib>:"CTRE_Phoenix_MotorControl_Set.vi"("Output"=w314, "Control Mode"=w315, "PhoenixMotorControlDevRef"=w313) -> ()  [unwired: 7 in, 2 out]
    }
    frame "New Testing Output" {
      w318 = T9 0 items=["PercentOutput"=0, "Position"=1, "Velocity"=2, "Current"=3, "Follower"=5, "MotionProfile"=6, "MotionMagic"=7, "MotionProfileArc"=10, "Disabled"=15] ("Control Mode")
      n167 = call <vilib>:"CTRE_Phoenix_MotorControl_Set.vi"("Output"=w316, "Control Mode"=w318, "PhoenixMotorControlDevRef"=w317) -> ()  [unwired: 7 in, 2 out]
    }
  }
  n168 = global read "GlobalDrivebase.vi" "REF_Shifter_2"() -> (w3:string)
  n169 = global read "GlobalDrivebase.vi" "REF_Shifter_0"() -> (w5:string)
  n170 = global read "GlobalDrivebase.vi" "REF_Shifter_3"() -> (w2:string)
  n171 = global read "GlobalDrivebase.vi" "REF_Shifter_1"() -> (w4:string)
  n172 = Equal?(x="Drive_3_(p)" ("Actuator_Name"), y=w138) -> (x = y?=w137:bool)
  n173 = Equal?(x="Drive_2_(p)" ("Actuator_Name"), y=w100) -> (x = y?=w99:bool)
  n174 = Equal?(x="Drive_0_(p)" ("Actuator_Name"), y=w86) -> (x = y?=w85:bool)
  n175 = Equal?(x="Drive_1_(p)" ("Actuator_Name"), y=w93) -> (x = y?=w92:bool)
  n176 = call-poly "GetRefNumFast.vi"("RefNum Name"=w2) -> ("Device Reference"=w103:T11)  [unwired: 5 in, 1 out]
  n177 = call-poly "TestActuatorInterlock.vi"("Normal Output"=w57, "Override Actuator Bypass"=w137, "Actuator Name"="Swerve_3_Shifter_(b)" ("Actuator_Name")) -> ("Interlocked Output"=w104:bool, "Output Mode"=w105:T10)  [unwired: 2 in]
  n178 = call-poly "GetRefNumFast.vi"("RefNum Name"=w3) -> ("Device Reference"=w96:T11)  [unwired: 5 in, 1 out]
  n179 = call-poly "TestActuatorInterlock.vi"("Normal Output"=w58, "Override Actuator Bypass"=w99, "Actuator Name"="Swerve_2_Shifter_(b)" ("Actuator_Name")) -> ("Interlocked Output"=w97:bool, "Output Mode"=w98:T10)  [unwired: 2 in]
  n180 = call-poly "GetRefNumFast.vi"("RefNum Name"=w5) -> ("Device Reference"=w82:T11)  [unwired: 5 in, 1 out]
  n181 = call-poly "TestActuatorInterlock.vi"("Normal Output"=w60, "Override Actuator Bypass"=w85, "Actuator Name"="Swerve_0_Shifter_(b)" ("Actuator_Name")) -> ("Interlocked Output"=w83:bool, "Output Mode"=w84:T10)  [unwired: 2 in]
  n182 = call-poly "GetRefNumFast.vi"("RefNum Name"=w4) -> ("Device Reference"=w89:T11)  [unwired: 5 in, 1 out]
  n183 = call-poly "TestActuatorInterlock.vi"("Normal Output"=w59, "Override Actuator Bypass"=w92, "Actuator Name"="Swerve_1_Shifter_(b)" ("Actuator_Name")) -> ("Interlocked Output"=w90:bool, "Output Mode"=w91:T10)  [unwired: 2 in]
  n184 = case shown="\"New Normal Output\"" w105 {
    tunnel: w104 -> [_ w320 w325]
    tunnel: w103 -> [_ w319 w324]
    frame "No Changed Output", Default {
    }
    frame "New Normal Output" {
      n185 = Select(t=WPI_SolenoidValue."Reverse" ("Value"), s=w320, f=WPI_SolenoidValue."Forward" ("Value")) -> (s? t:f=w321:T13)
      n186 = call-poly <vilib>:"WPI_SolenoidSet.vi"("Value"=w321, "SolenoidDevRef"=w319) -> ()  [unwired: 8 in, 2 out]
    }
    frame "New Testing Output" {
      n187 = Select(t=WPI_SolenoidValue."Reverse" ("Value"), s=w325, f=WPI_SolenoidValue."Forward" ("Value")) -> (s? t:f=w328:T13)
      n188 = call-poly <vilib>:"WPI_SolenoidSet.vi"("Value"=w328, "SolenoidDevRef"=w324) -> ()  [unwired: 8 in, 2 out]
    }
  }
  n189 = case shown="\"New Normal Output\"" w98 {
    tunnel: w97 -> [_ w330 w335]
    tunnel: w96 -> [_ w329 w334]
    frame "No Changed Output", Default {
    }
    frame "New Normal Output" {
      n190 = Select(t=WPI_SolenoidValue."Reverse" ("Value"), s=w330, f=WPI_SolenoidValue."Forward" ("Value")) -> (s? t:f=w331:T13)
      n191 = call-poly <vilib>:"WPI_SolenoidSet.vi"("Value"=w331, "SolenoidDevRef"=w329) -> ()  [unwired: 8 in, 2 out]
    }
    frame "New Testing Output" {
      n192 = Select(t=WPI_SolenoidValue."Reverse" ("Value"), s=w335, f=WPI_SolenoidValue."Forward" ("Value")) -> (s? t:f=w338:T13)
      n193 = call-poly <vilib>:"WPI_SolenoidSet.vi"("Value"=w338, "SolenoidDevRef"=w334) -> ()  [unwired: 8 in, 2 out]
    }
  }
  n194 = case shown="\"New Normal Output\"" w84 {
    tunnel: w83 -> [_ w340 w345]
    tunnel: w82 -> [_ w339 w344]
    frame "No Changed Output", Default {
    }
    frame "New Normal Output" {
      n195 = Select(t=WPI_SolenoidValue."Reverse" ("Value"), s=w340, f=WPI_SolenoidValue."Forward" ("Value")) -> (s? t:f=w341:T13)
      n196 = call-poly <vilib>:"WPI_SolenoidSet.vi"("Value"=w341, "SolenoidDevRef"=w339) -> ()  [unwired: 8 in, 2 out]
    }
    frame "New Testing Output" {
      n197 = Select(t=WPI_SolenoidValue."Reverse" ("Value"), s=w345, f=WPI_SolenoidValue."Forward" ("Value")) -> (s? t:f=w348:T13)
      n198 = call-poly <vilib>:"WPI_SolenoidSet.vi"("Value"=w348, "SolenoidDevRef"=w344) -> ()  [unwired: 8 in, 2 out]
    }
  }
  n199 = case shown="\"New Normal Output\"" w91 {
    tunnel: w90 -> [_ w350 w355]
    tunnel: w89 -> [_ w349 w354]
    frame "No Changed Output", Default {
    }
    frame "New Normal Output" {
      n200 = Select(t=WPI_SolenoidValue."Reverse" ("Value"), s=w350, f=WPI_SolenoidValue."Forward" ("Value")) -> (s? t:f=w351:T13)
      n201 = call-poly <vilib>:"WPI_SolenoidSet.vi"("Value"=w351, "SolenoidDevRef"=w349) -> ()  [unwired: 8 in, 2 out]
    }
    frame "New Testing Output" {
      n202 = Select(t=WPI_SolenoidValue."Reverse" ("Value"), s=w355, f=WPI_SolenoidValue."Forward" ("Value")) -> (s? t:f=w358:T13)
      n203 = call-poly <vilib>:"WPI_SolenoidSet.vi"("Value"=w358, "SolenoidDevRef"=w354) -> ()  [unwired: 8 in, 2 out]
    }
  }
